vi "Write Spectrometer Driver.lvclass.vi"(8 "error in (no error)":errorcluster, 10 "Spectrometer Driver.lvclass":refnum<class "Spectrometer Driver.lvclass">, 11 "Spectrometer in":refnum<class "Spectrometer.lvclass">) -> (0 "error out":errorcluster, 3 "Spectrometer out":refnum<class "Spectrometer.lvclass">)   [LabVIEW 2018, in "Spectrometer.lvclass"]
uses:
  Spectrometer.lvclass
  C:/github/LabActor/Instrument Actor/Instrument Actor.lvclass
  NHMFL_Core/Libraries/Instruments/Spectrometer Driver/Spectrometer Driver.lvclass
  C:/github/NHMFL_Core/Libraries/Instruments/Instrument Driver/Instrument Driver.lvclass
  Instrument Actor/Instrument Actor.lvclass/Instrument Actor.ctl
  Instrument Actor/Write Instrument driver.vi
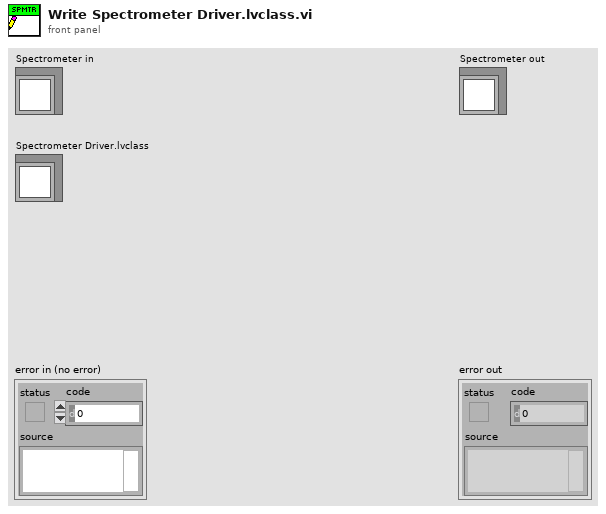
[diagram p1: front panel]
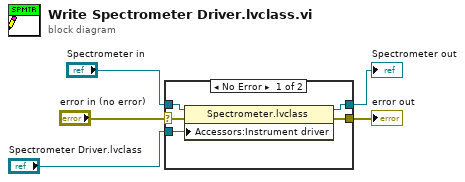
[diagram p0: block diagram]
diagram:
  n1 = case shown="No Error" "error in (no error)" {
    selector: "error in (no error)" -> [w10 w11]
    tunnel: [w9 w11] -> w4
    tunnel: [w7 w12] -> w2
    tunnel: "Spectrometer in" -> [w8 w12]
    tunnel: "Spectrometer Driver.lvclass" -> [w6 _]
    frame No Error {
      n2 = property class="Spectrometer.lvclass"(reference=w8, error in=w10, "Accessors:Instrument driver"=w6) -> (reference out=w7:refnum<class "Spectrometer.lvclass">, error out=w9:errorcluster)
    }
    frame Error {
    }
  }
  "error out" <- w4
  "Spectrometer out" <- w2
